vi "detector_acquire_generic_data.vi"(8 "error in (no error)":errorcluster, 11 "lightfield_class in":refnum<class "lightfield_class.lvclass">) -> (0 "error out":errorcluster, 2 "image_data":T1, 3 "lightfield_class out":refnum<class "lightfield_class.lvclass">)   [LabVIEW 2015, in "lightfield_class.lvclass"]
uses:
  lightfield_class.lvclass
  Experiment/experiment_panel/2d_scan/detector_data_tdef.ctl
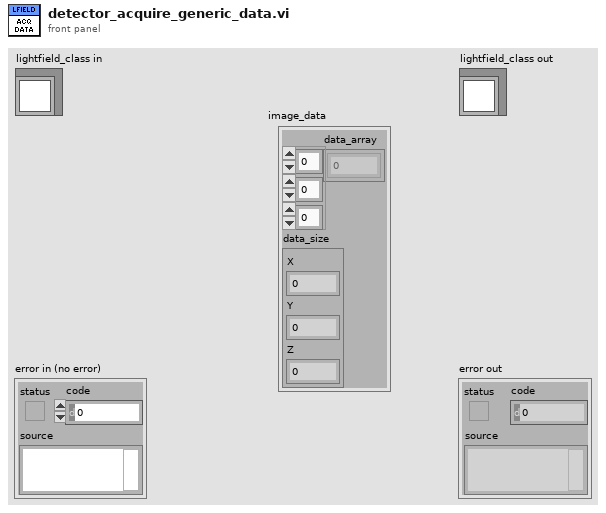
[diagram p1: front panel]
types:
  T1 = typedef "detector_data_tdef.ctl" = cluster{"data_array":dbl[][][], "data_size":cluster{"X":i32, "Y":i32, "Z":i32}}
  T2 = cluster{"Image":dbl[][][], "Frame Size":cluster{"F":i32, "Y":i32, "X":i32}}
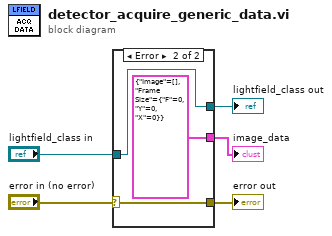
[diagram p0: block diagram]
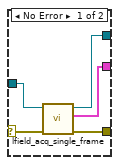
[diagram p2: hidden frame]
diagram:
  n1 = case shown="Error" "error in (no error)" {
    selector: "error in (no error)" -> [w10 w11]
    tunnel: [w9 w11] -> w4
    tunnel: "lightfield_class in" -> [w8 w13]
    tunnel: [w7 w13] -> w2
    tunnel: [w6 T2 {"Image"=[], "Frame Size"={"F"=0, "Y"=0, "X"=0}} ("image_data")] -> w1
    frame No Error {
      n2 = call "lfield_acq_single_frame.vi"("error in (no error)"=w10, "lightfield_class in"=w8) -> ("error out"=w9:errorcluster, "image_data"=w6:T2, "lightfield_class out"=w7:refnum<class "lightfield_class.lvclass">)  [unwired: 7 in]
    }
    frame Error {
    }
  }
  "error out" <- w4
  "lightfield_class out" <- w2
  "image_data" <- w1
